vi "Act.vi"(8 "error in (no error)":errorcluster, 9 "VI Refnum in":refnum<vi>, 10 "Flex Msg type":refnum<class "Flex Msg.lvclass">, 11 "Set Controls in":refnum<class "Set Controls.lvclass">) -> (0 "error out":errorcluster, 1 "Await user action?":bool, 3 "Set Controls out":refnum<class "Set Controls.lvclass">)   [LabVIEW 2020, in "Msg.lvlib" / "Set Controls.lvclass"]
doc: "Set the front panel control data and does not wait for user action."
uses:
  Set Controls.lvclass
  Flex Msg.lvclass
  Set Controls.lvclass/Set Controls.ctl
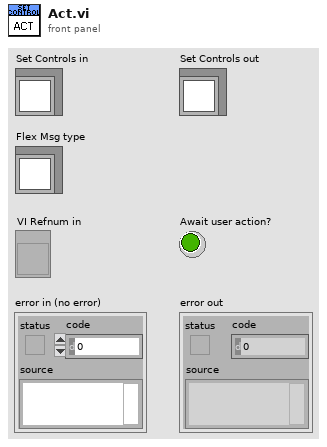
[diagram p1: front panel]
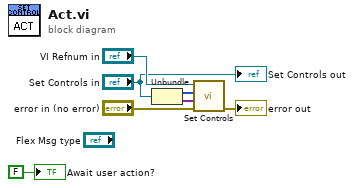
[diagram p0: block diagram]
diagram:
  n1 = Unbundle("Set Controls in") -> (w3:i32[], w2:variant[])
  n2 = call "Set Controls.vi"("error in (no error)"="error in (no error)", "data values"=w2, "control indexes"=w3, "VI Refnum in"="VI Refnum in") -> ("error out"=→"error out":errorcluster)  [unwired: 7 in]
  "Set Controls out" <- "Set Controls in"
  "Await user action?" <- FALSE ("Await user action?")
